vi "Area.vi"(8 "error in":errorcluster, 11 "Square in":refnum<class "Square.lvclass">) -> (0 "error out":errorcluster, 2 "area":dbl, 3 "Square out":refnum<class "Square.lvclass">)   [LabVIEW 2015, in "Square.lvclass"]
uses:
  Square.lvclass
  Square.lvclass/Square.ctl
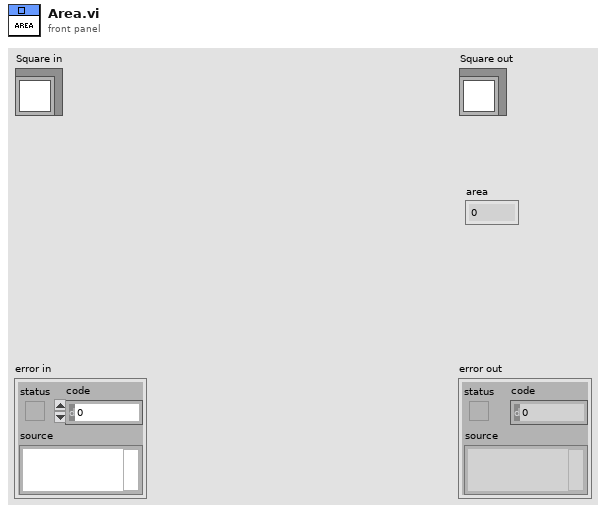
[diagram p1: front panel]
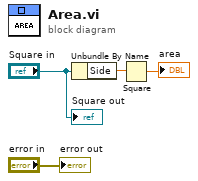
[diagram p0: block diagram]
diagram:
  n1 = Unbundle By Name("Square in") -> ("Side"=w4:dbl)
  n2 = Square(x=w4) -> (x^2=→"area":dbl)
  "error out" <- "error in"
  "Square out" <- "Square in"
